vi "Get Oven Type.vi"(8 "Error In":errorcluster, 11 "reference in":refnum<class "Recipe Step.lvclass">) -> (0 "Error Out":errorcluster, 1 "Oven Type":refnum<class "Oven Actor.lvclass">, 2 "Oven Type":string(combo), 3 "reference out":refnum<class "Recipe Step.lvclass">)   [LabVIEW 2024, in "Recipe Step.lvclass"]
uses:
  Recipe Step.lvclass
  Recipe Step.lvclass/Recipe Step.ctl
  Oven Actor/Direct Oven/Direct Oven.lvclass
  Oven Actor/Ramp Oven/Ramp Oven.lvclass
  C:/Users/burakkorkmaz/Desktop/Leveling/repo/Oven Actor/Oven Actor/Oven Actor.lvclass
  C:/Program Files/National Instruments/LabVIEW 2024/vi.lib/ActorFramework/Actor/Actor.lvclass
  C:/Users/burakkorkmaz/Desktop/Leveling/repo/Oven Actor/Direct Oven/Direct Oven.lvclass
  C:/Users/burakkorkmaz/Desktop/Leveling/repo/Oven Actor/Ramp Oven/Ramp Oven.lvclass
  Oven Actor/Oven Actor/Oven Actor.lvclass
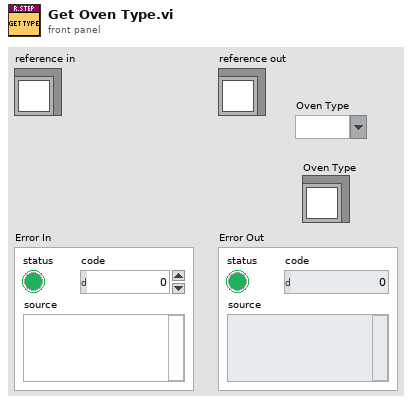
[diagram p1: front panel]
types:
  T1 = typedef "Recipe Step.lvclass/ObjectAttributes.ctl" = cluster{"Step Data":cluster{"Fire (%)":dbl, "Duration (s)":dbl, "Oven Type":string}}
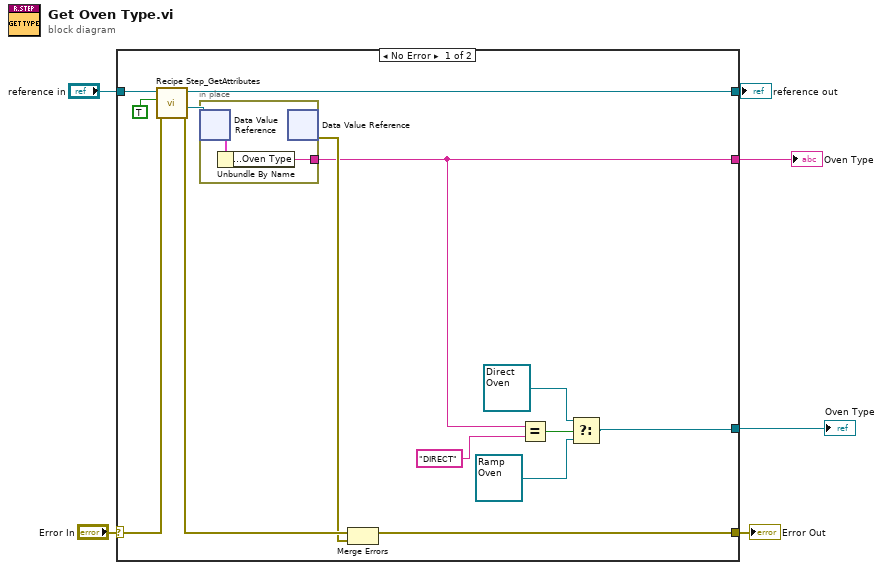
[diagram p0: block diagram]
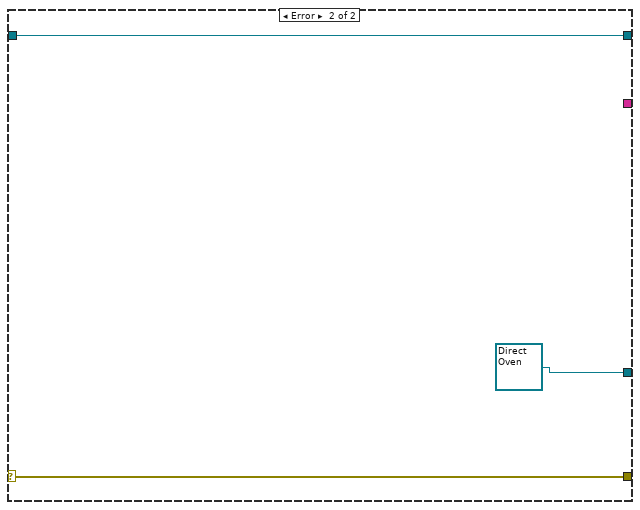
[diagram p2: hidden frame]
diagram:
  n1 = case shown="No Error" "Error In" {
    selector: "Error In" -> [w20 w25]
    tunnel: [w18 w25] -> w5
    tunnel: [w15 w24] -> w3
    tunnel: "reference in" -> [w16 w24]
    tunnel: [w8 _] -> w2
    tunnel: [w7 refnum<class "Direct Oven.lvclass"> refnum ("Oven Actor.lvlib:Direct Oven.lvclass")] -> w1
    frame No Error {
      n2 = call "Recipe Step_GetAttributes.vi"("Error In"=w20, "OnlyGetDvrReference(False)"=TRUE, "reference in"=w16) -> ("Error Out"=w19:errorcluster, "DataRef"=w13:refnum<data-value>, "reference out"=w15:refnum<class "Recipe Step.lvclass">)  [unwired: 5 in, 1 out]
      n3 = in-place {
        in-place-border: [w22] -> w8
        n4 = in-place-dvr #1(w13) -> (w21:T1)  [unwired: 1 out]
        n5 = Unbundle By Name(w21) -> ("Step Data.Oven Type"=w22:string)
        n6 = in-place-dvr #1() -> (w17:errorcluster)  [unwired: 1 in, 1 out]
      }
      n7 = Merge Errors(w19, w17) -> (w18:errorcluster)
      n8 = Equal?(x=w8, y="DIRECT") -> (x = y?=w12:bool)
      n9 = Select(t=refnum<class "Direct Oven.lvclass"> refnum ("Oven Actor.lvlib:Direct Oven.lvclass"), s=w12, f=refnum<class "Ramp Oven.lvclass"> refnum ("Oven Actor.lvlib:Ramp Oven.lvclass")) -> (s? t:f=w7:refnum<class "Oven Actor.lvclass">)
    }
    frame Error {
    }
  }
  "Error Out" <- w5
  "reference out" <- w3
  "Oven Type" <- w2
  "Oven Type" <- w1
